vi "Unscramble_Multiplex_chs.vi"(1 "No of Samples per multiplexer clock":i32=2, 2 "Multiplex Ch No":i16[](array[numeric]), 3 "Channel Numbers":i16[](array[numeric]), 4 "Voltages":dbl[][](array[numeric])) -> (0 "Voltage by Req Ch":dbl[][](array[numeric]))   [LabVIEW 2022 SP3]
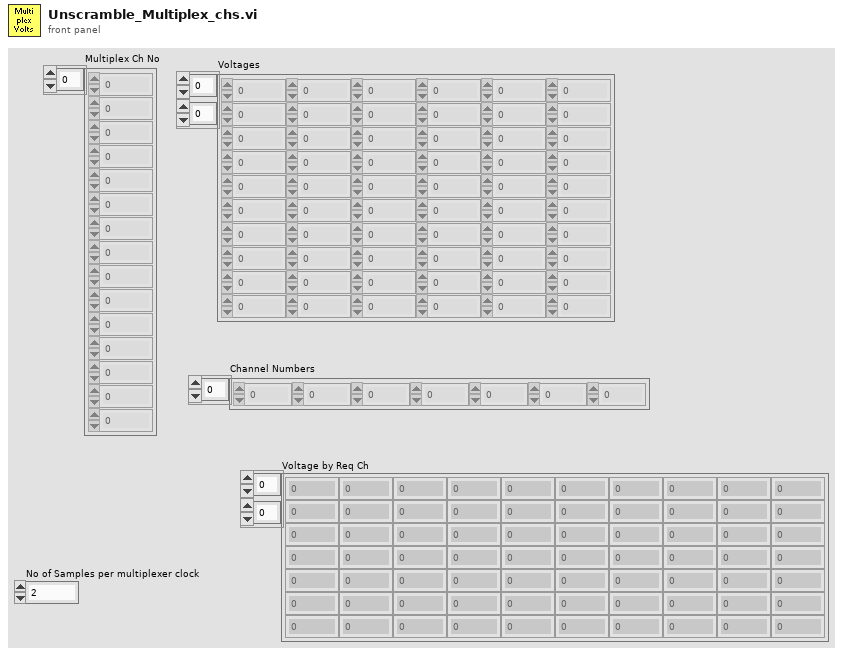
[diagram p1: front panel]
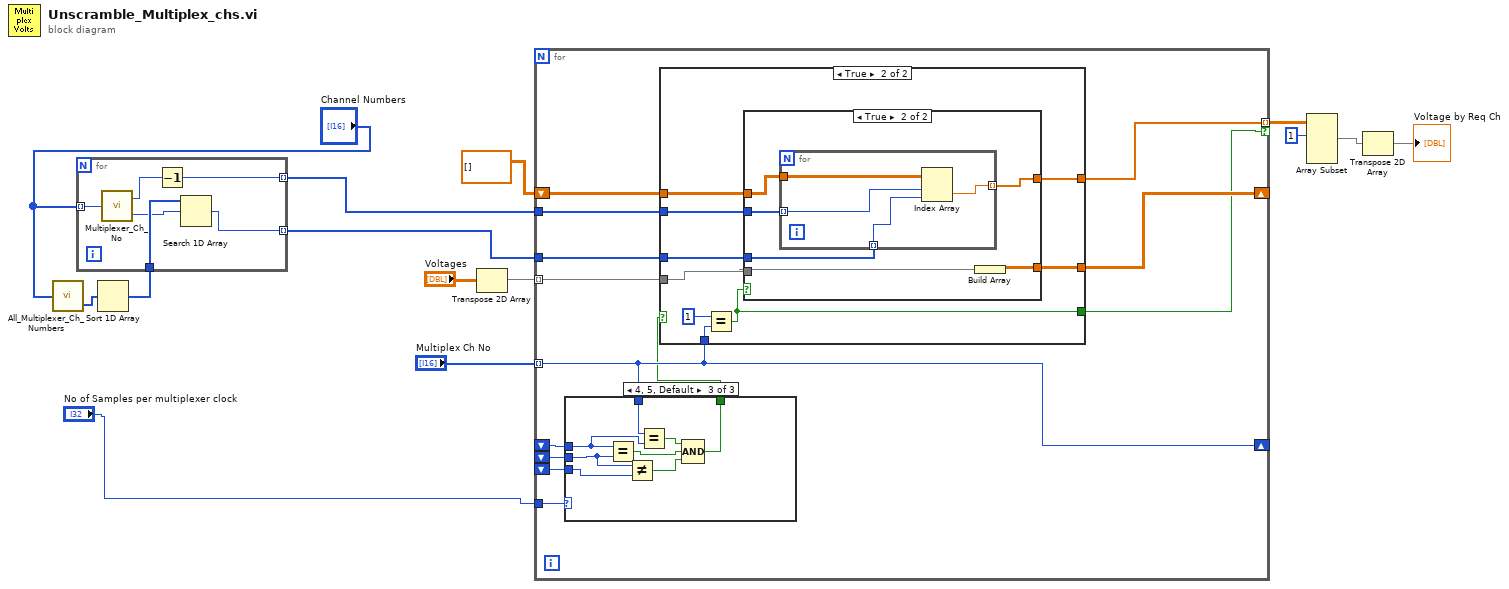
[diagram p0: block diagram]
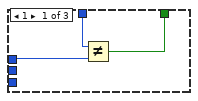
[diagram p2: hidden frame]
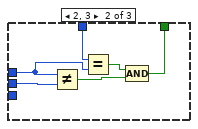
[diagram p3: hidden frame]
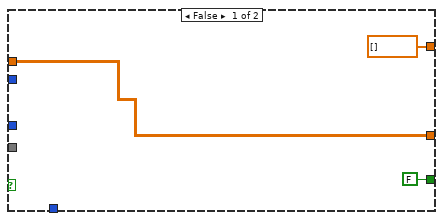
[diagram p4: hidden frame]
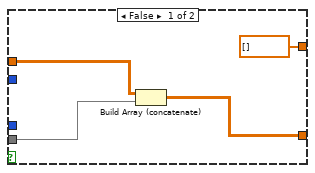
[diagram p5: hidden frame]
diagram:
  n1 = call "All_Multiplexer_Ch_Numbers.vi"("Channel Numbers"="Channel Numbers") -> ("ADC Ch No"=w2:i16[])  [unwired: 1 out]
  n2 = Sort 1D Array(array=w2) -> (sorted array=w3:i16[])
  n3 = for {
    tunnel: "Channel Numbers" -> [w20] mode=indexing
    tunnel: w3 -> [w19]
    tunnel: [w16] -> w5 mode=indexing
    tunnel: [w15] -> w4 mode=indexing
    n4 = call "Multiplexer_Ch_No.vi"("Channel Number"=w20) -> ("Multiplexer Ch No"=w17:i16, "ADC Ch No"=w18:i16)
    n5 = Decrement(x=w17) -> (x-1=w16:i16)
    n6 = Search 1D Array(1D array=w19, element=w18) -> (index of element=w15:i32)  [unwired: 1 in]
  }
  n7 = Transpose 2D Array(2D array="Voltages") -> (transposed array=w9:dbl[][])
  n8 = for {
    tunnel: "Multiplex Ch No" -> [w32] mode=indexing
    shift-right: [w32] -> _
    shift-left: _ -> [w33]
    shift-left: _ -> [w23]
    shift-right: [w29] -> _
    shift-left: dbl[][] [] -> [w30]
    tunnel: w9 -> [w31] mode=indexing
    tunnel: [w27] -> w12 mode=indexing if=w26
    tunnel: w5 -> [w25]
    tunnel: w4 -> [w24]
    shift-left: _ -> [w22]
    tunnel: "No of Samples per multiplexer clock" -> [w21]
    n9 = case shown="4, 5, Default" w21 {
      tunnel: w33 -> [w36 w42 w50]
      tunnel: w32 -> [w35 w39 w47]
      tunnel: [w34 w38 w46] -> w28
      tunnel: w23 -> [_ w37 w45]
      tunnel: w22 -> [_ _ w44]
      frame 1 {
        n10 = Not Equal?(x=w35, y=w36) -> (x != y?=w34:bool)
      }
      frame 2, 3 {
        n11 = Not Equal?(x=w42, y=w37) -> (x != y?=w40:bool)
        n12 = Equal?(x=w39, y=w42) -> (x = y?=w41:bool)
        n13 = Compound Arithmetic op=AND(w41, w40) -> (w38:bool)
      }
      frame 4, 5, Default {
        n14 = Equal?(x=w50, y=w45) -> (x = y?=w48:bool)
        n15 = Not Equal?(x=w45, y=w44) -> (x != y?=w43:bool)
        n16 = Equal?(x=w47, y=w50) -> (x = y?=w49:bool)
        n17 = Compound Arithmetic op=AND(w49, w48, w43) -> (w46:bool)
      }
    }
    n18 = case shown="True" w28 {
      tunnel: w32 -> [_ w59]
      tunnel: w31 -> [_ w62]
      tunnel: w30 -> [w53 w61]
      tunnel: [w53 w60] -> w29
      tunnel: [dbl[] [] w57] -> w27
      tunnel: [FALSE w56] -> w26
      tunnel: w25 -> [_ w55]
      tunnel: w24 -> [_ w54]
      frame False {
      }
      frame True {
        n19 = Equal?(x=i16 1, y=w59) -> (x = y?=w56:bool)
        n20 = case shown="True" w56 {
          tunnel: w62 -> [w66 w72]
          tunnel: w61 -> [w65 w70]
          tunnel: [w64 w71] -> w60
          tunnel: [dbl[] [] w69] -> w57
          tunnel: w55 -> [_ w68]
          tunnel: w54 -> [_ w67]
          frame False {
            n21 = Build Array (concatenate)(w65, w66) -> (w64:dbl[][])
          }
          frame True {
            n22 = for {
              tunnel: w70 -> [w76]
              tunnel: [w75] -> w69 mode=indexing
              tunnel: w68 -> [w74] mode=indexing
              tunnel: w67 -> [w73] mode=indexing
              n23 = Index Array(array=w76, index (row)=w74, index (col)=w73) -> (element=w75:dbl)
            }
            n24 = Build Array(w72) -> (w71:dbl[][])
          }
        }
      }
    }
  }
  n25 = Array Subset(array=w12, index (row)=1 ("index")) -> (w8:dbl[][])  [unwired: 3 in]
  n26 = Transpose 2D Array(2D array=w8) -> (transposed array=→"Voltage by Req Ch":dbl[][])
